vi "Zebra 串口.vi"(8 "error in":errorcluster, 9 "write buffer":string, 10 "波特率":u32=9600, 11 "VISA 名称":refnum<visa-resource-name>) -> (0 "error out":errorcluster)   [LabVIEW 2016]
uses:
  <vilib>/Instr/_visa.llb/VISA Configure Serial Port (Instr).vi
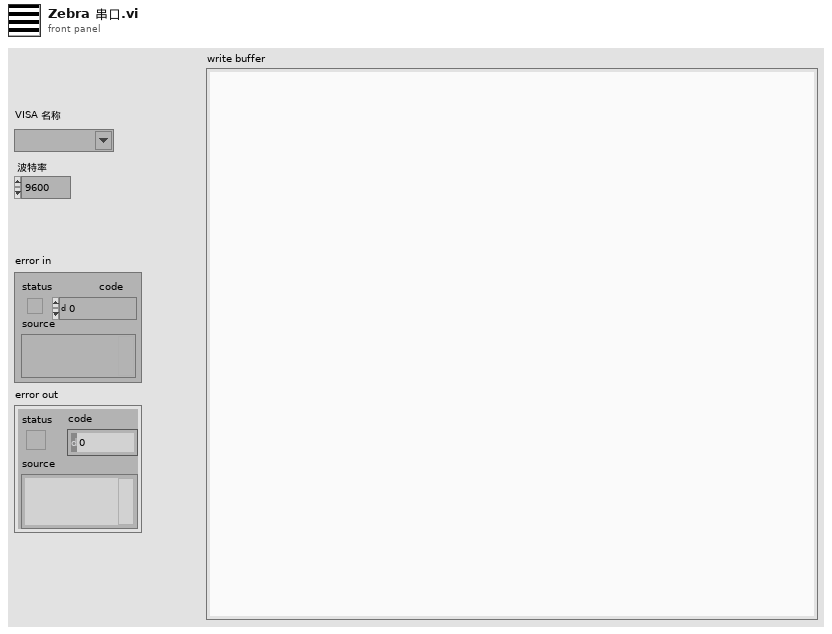
[diagram p1: front panel]
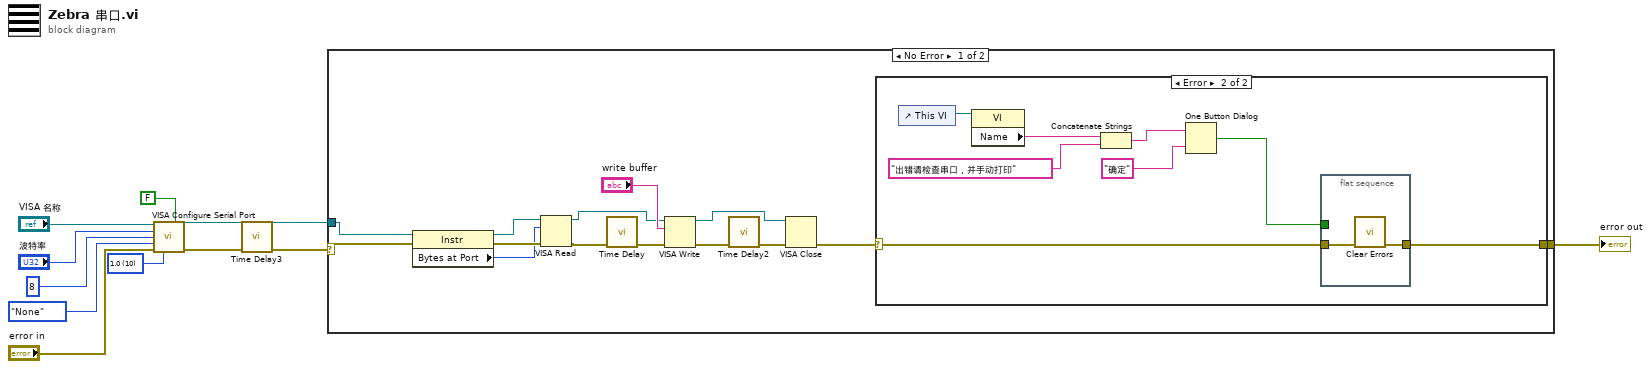
[diagram p0: block diagram]
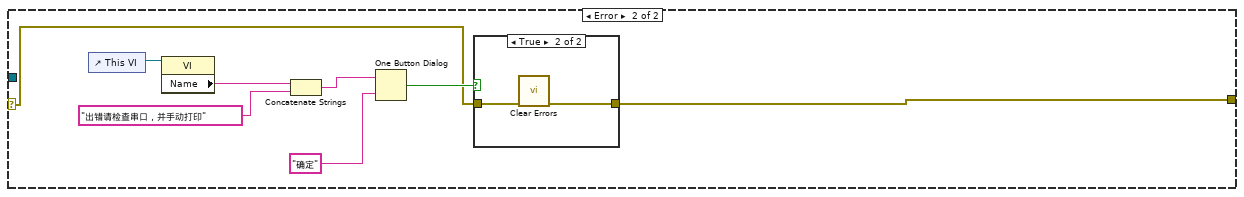
[diagram p3: hidden frame]
diagram:
  w11 = u16 10 items=["1.0"=10, "1.5"=15, "2.0"=20] ("stop bits (10: 1 bit)")
  n1 = call-poly "VISA Configure Serial Port"("VISA resource name"="VISA 名称", "Enable Termination\nChar (T)"=FALSE ("Enable Termination\nChar (T)"), "baud rate (9600)"="波特率", "data bits (8)"=u16 8, "parity (0:none)"=enum16{"None", "Odd", "Even", "Mark", "Space"}."None", "error in (no error)"="error in", "stop bits (10: 1 bit)"=w11) -> ("VISA resource name out"=w5:refnum<visa-resource-name>, "error out"=w2:errorcluster)  [unwired: 7 in]
  n2 = call "Time Delay3"("error in (no error)"=w2) -> ("error out"=w1:errorcluster)  [unwired: 10 in]
  n3 = case shown="No Error" w1 {
    selector: w1 -> [w17 w38]
    tunnel: w5 -> [w18 _]
    tunnel: [w12 w37] -> w3
    frame No Error {
      n4 = property class="Instr"(reference=w18, error in=w17) -> (reference out=w19:refnum<visa-resource-name>, error out=w20:errorcluster, "Bytes at Port"=w14:u32)
      n5 = VISA Read(VISA resource name=w19, byte count=w14, error in (no error)=w20) -> (VISA resource name out=w16:refnum<visa-resource-name>, error out=w15:errorcluster)  [unwired: 2 out]
      n6 = call "Time Delay"("error in (no error)"=w15) -> ("error out"=w25:errorcluster)  [unwired: 10 in]
      n7 = VISA Write(VISA resource name=w16, write buffer="write buffer", error in (no error)=w25) -> (VISA resource name out=w22:refnum<visa-resource-name>, error out=w24:errorcluster)  [unwired: 1 out]
      n8 = call "Time Delay2"("error in (no error)"=w24) -> ("error out"=w23:errorcluster)  [unwired: 10 in]
      n9 = VISA Close(VISA resource name=w22, error in (no error)=w23) -> (error out=w13:errorcluster)
      n10 = case shown="Error" w13 {
        selector: w13 -> [w26 w29]
        tunnel: [w26 w28] -> w12
        frame No Error {
        }
        frame Error {
          n11 = control-ref of="This VI"() -> (w34:refnum<vi>)
          n12 = property class="VI"(reference=w34) -> ("Name"=w33:string)  [unwired: 1 in, 2 out]
          n13 = Concatenate Strings(w33, "出错请检查串口，并手动打印" ("string")) -> (w31:string)
          n14 = One Button Dialog(message=w31, button name ("OK")="确定") -> (true=w27:bool)
          n15 = flat-sequence {
            tunnel: w29 -> [w36]
            tunnel: [w35] -> w28
            tunnel: w27 -> [_]
            frame #0 {
              n16 = call <vilib>:"Clear Errors.vi"("error in (no error)"=w36) -> ("error out"=w35:errorcluster)  [unwired: 5 in, 1 out]
            }
          }
        }
      }
    }
    frame Error {
      n17 = control-ref of="This VI"() -> (w44:refnum<vi>)
      n18 = property class="VI"(reference=w44) -> ("Name"=w43:string)  [unwired: 1 in, 2 out]
      n19 = Concatenate Strings(w43, "出错请检查串口，并手动打印" ("string")) -> (w41:string)
      n20 = One Button Dialog(message=w41, button name ("OK")="确定") -> (true=w39:bool)
      n21 = case shown="True" w39 {
        tunnel: w38 -> [w45 w47]
        tunnel: [w45 w46] -> w37
        frame False {
        }
        frame True {
          n22 = call <vilib>:"Clear Errors.vi"("error in (no error)"=w47) -> ("error out"=w46:errorcluster)  [unwired: 5 in, 1 out]
        }
      }
    }
  }
  "error out" <- w3
